vi "Unflatten vers.vi"(8 "error in (no error)":errorcluster, 11 "Data in":string) -> (0 "error out":errorcluster, 3 "vers":T1 {"Flags" format="%04x"})   [LabVIEW 2018, in "VI-Hacker.lvlib"]
uses:
  VI-Hacker.lvlib
  <vilib>/Utility/error.llb/Error Cluster From Error Code.vi
  <vilib>/ErrorRing/Error Ring.xnode
  TypeDefs/Block vers.ctl
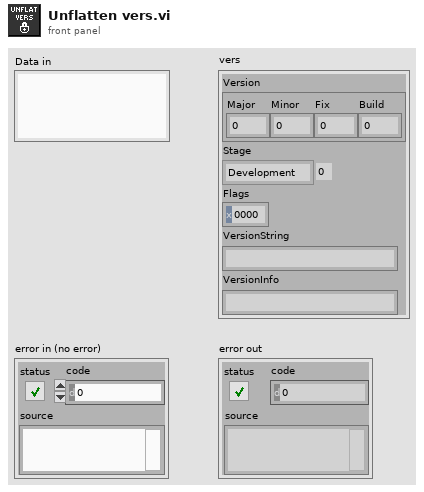
[diagram p1: front panel]
types:
  T1 = typedef "VI-Hacker.lvlib/Block vers.ctl" = cluster{"Version":cluster{"Major":u8, "Minor":u8, "Fix":u8, "Build":u8}, "Stage":enum8{"Development", "Alpha", "Beta", "Release"}, "Flags":u16, "VersionString":string, "VersionInfo":string}
  T2 = cluster{"Version":u32, "Flags":u16, "VerStrLen":u8}
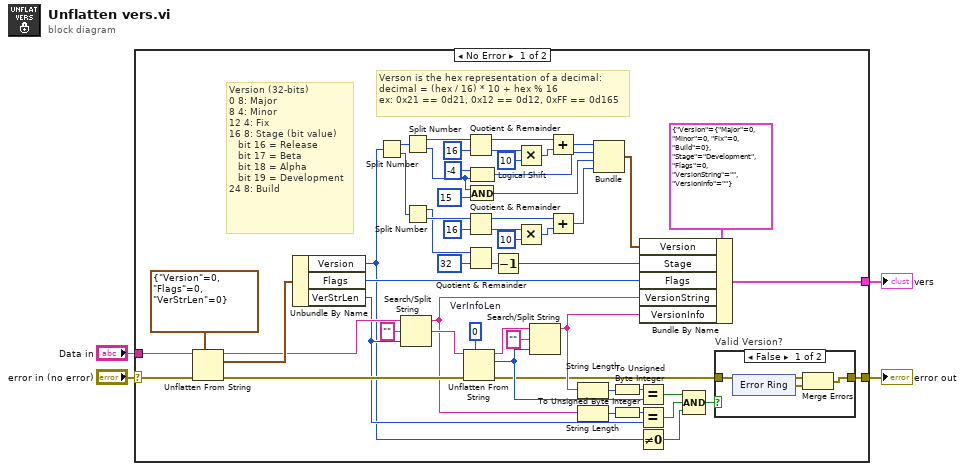
[diagram p0: block diagram]
diagram:
  n1 = case shown="No Error" "error in (no error)" {
    selector: "error in (no error)" -> [w7 w69]
    tunnel: [w59 _] -> w4
    tunnel: [w58 w69] -> w2
    tunnel: "Data in" -> [w6 _]
    frame No Error {
      w55 = u8 0  # VerInfoLen
      # "Verson is the hex representation of a decimal:\ndecimal = (hex / 16) * 10 + hex % 16\nex: 0x21 == 0d21, 0x12 == 0d12, 0xFF == 0d165"
      # "Version (32-bits)\n0 8: Major\n8 4: Minor\n12 4: Fix\n16 8: Stage (bit value)\n   bit 16 = Release\n   bit 17 = Beta\n   bit 18 = Alpha\n   bit 19 = Development\n24 8: Build"
      n2 = Unflatten From String(type=T2 {"Version"=0, "Flags"=0, "VerStrLen"=0} ("vers"), binary string=w6, error in (no error)=w7) -> (rest of the binary string=w53:string, value=w56:T2, error out=w54:errorcluster)  [unwired: 2 in]
      n3 = Unbundle By Name(w56) -> ("Version"=w9:u32, "Flags"=w22:u16, "VerStrLen"=w19:u8)
      n4 = Split Number(x=w9) -> (hi(x)=w47:u16, lo(x)=w48:u16)
      n5 = Search/Split String(string=w53, search string/char (-)="", offset (0)=w19) -> (substring before match=w21:string, match + rest of string=w50:string)  [unwired: 1 out]
      n6 = Split Number(x=w47) -> (hi(x)=w46:u8, lo(x)=w30:u8)
      n7 = Split Number(x=w48) -> (hi(x)=w26:u8, lo(x)=w35:u8)
      n8 = Unflatten From String(type=w55, binary string=w50, error in (no error)=w54) -> (rest of the binary string=w49:string, value=w14:u8, error out=w11:errorcluster)  [unwired: 2 in]
      n9 = Quotient & Remainder(x=w46, y=u8 16) -> (x-y*floor(x/y)=w41:u8, floor(x/y)=w44:u8)
      n10 = Quotient & Remainder(x=w35, y=u8 16) -> (x-y*floor(x/y)=w40:u8, floor(x/y)=w37:u8)
      n11 = Quotient & Remainder(x=w26, y=u8 32) -> (floor(x/y)=w25:u8)  [unwired: 1 out]
      n12 = Logical Shift(y=i16 -4, x=w30) -> (x << y=w28:u8)
      n13 = And(x=w30, y=u8 15) -> (x .and. y?=w31:u8)
      n14 = Decrement(x=w25) -> (x-1=w23:u8)
      n15 = Multiply(x=w44, y=u8 10) -> (x*y=w42:u8)
      n16 = Multiply(x=w37, y=u8 10) -> (x*y=w39:u8)
      n17 = Search/Split String(string=w49, search string/char (-)="", offset (0)=w14) -> (substring before match=w15:string)  [unwired: 2 out]
      n18 = Add(x=w41, y=w42) -> (x+y=w34:u8)
      n19 = Add(x=w40, y=w39) -> (x+y=w33:u8)
      n20 = String Length(string=w15) -> (length=w16:i32)
      n21 = String Length(string=w21) -> (length=w20:i32)
      n22 = Bundle(w34, w28, w31, w33) -> (w24:cluster{u8, u8, u8, u8})  [unwired: 1 in]
      n23 = To Unsigned Byte Integer(number=w16) -> (unsigned 8bit integer=w17:u8)
      n24 = To Unsigned Byte Integer(number=w20) -> (unsigned 8bit integer=w18:u8)
      n25 = Equal?(x=w17, y=w14) -> (x = y?=w13:bool)
      n26 = Equal?(x=w18, y=w19) -> (x = y?=w12:bool)
      n27 = Not Equal To 0?(x=w9) -> (x != 0?=w8:bool)
      n28 = Bundle By Name(cluster=T1 {"Version"={"Major"=0, "Minor"=0, "Fix"=0, "Build"=0}, "Stage"=enum."Development", "Flags"=0, "VersionString"="", "VersionInfo"=""} ("vers"), "Version"=w24, "Stage"=w23, "Flags"=w22, "VersionString"=w21, "VersionInfo"=w15) -> (w59:T1)
      n29 = Compound Arithmetic op=AND(w13, w12, w8) -> (w10:bool)
      n30 = case "Valid Version?" shown="False" w10 {
        tunnel: [w61 w68] -> w58
        tunnel: w11 -> [w62 w68]
        frame False {
          n31 = xnode "Error Ring"() -> ("error out"=w60:errorcluster)
          n32 = Merge Errors(w62, w60) -> (w61:errorcluster)
        }
        frame True {
        }
      }
    }
    frame Error {
    }
  }
  "vers" <- w4
  "error out" <- w2
